vi "epics get uniformity.vi"(8 "error in":errorcluster, 11 "CA in":T2) -> (0 "error out":errorcluster, 1 "Status":bool, 2 "Values Out - String":string[](array[string]), 3 "Data Value Out":T3, 4 "PV Info":T1[](array[typedef]))   [LabVIEW 2022 SP3]
uses:
  Program Files/National Instruments/LabVIEW 2023/user.lib/calab/CaLab.lvlib
  Program Files/National Instruments/LabVIEW 2023/user.lib/calab/private/Get_PV.vi
  pectus/control/epics value.ctl
  271cf89c-c69d-42b5-ba05-be60b1157d68.vi
  pectus/control/ca cluster.ctl
  Program Files/National Instruments/LabVIEW 2023/user.lib/calab/PV Info.ctl
panel:
  out "Value out":variant
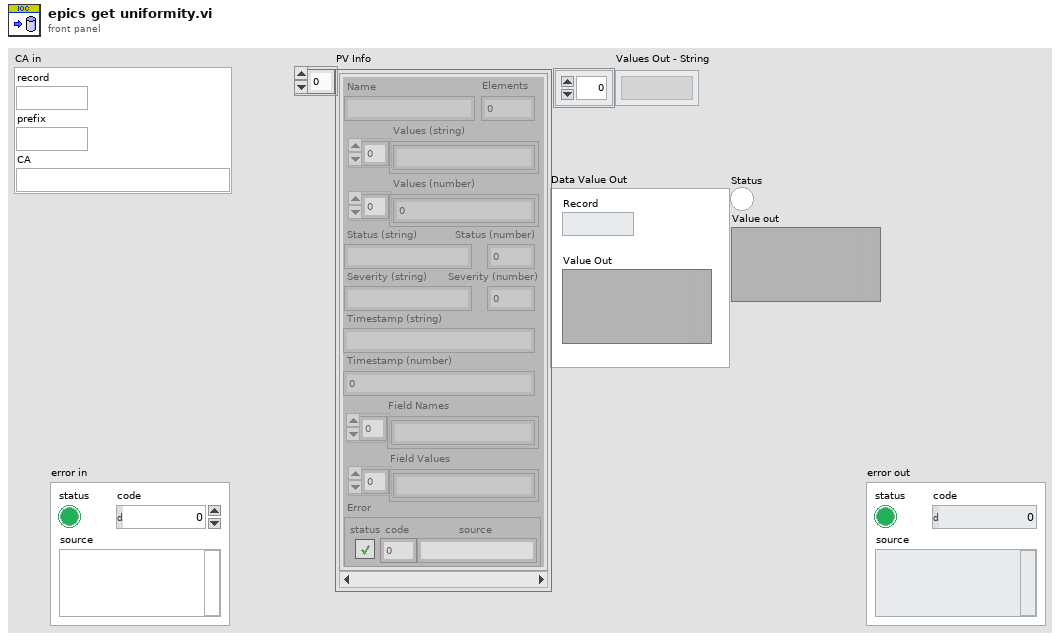
[diagram p1: front panel]
types:
  T1 = typedef "CaLab.lvlib/PV Info.ctl" = cluster{"Name":string, "Elements":i32, "Values (string)":string[], "Values (number)":dbl[], "Status (string)":string, "Status (number)":i16, "Severity (string)":string, "Severity (number)":i16, "Timestamp (string)":string, "Timestamp (number)":i32, "Field Names":string[], "Field Values":string[], "Error":errorcluster}
  T2 = typedef "ca cluster.ctl" = cluster{"record":string, "prefix":string, "CA":string}
  T3 = typedef "epics value.ctl" = cluster{"Record":string, "Value Out":variant}
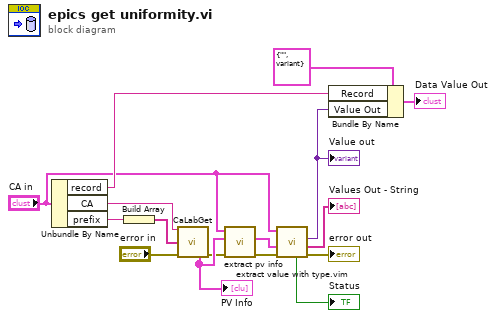
[diagram p0: block diagram]
diagram:
  n1 = Unbundle By Name("CA in") -> ("record"=w10:string, "CA"=w12:string, "prefix"=w11:string)
  n2 = Build Array(w11) -> (w16:string[])
  n3 = call-poly "CaLabGet.vi"("PV Name"=w12, "Field Names"=w16, "Error in (no error)"="error in") -> ("PV Info"=w8:T1[], "Error out"=w3:errorcluster)  [unwired: 6 in, 5 out]
  "PV Info" <- w8
  n4 = call "extract pv info.vi"("error in"=w3, "PV Info"=w8, "CA in"="CA in") -> ("error out"=w7:errorcluster, "PV Selected"=w6:T1)  [unwired: 7 in]
  n5 = call "extract value with type.vim"("error in"=w7, "PV Selected"=w6, "CA in"="CA in") -> ("error out"=→"error out":errorcluster, "Values Out - String"=→"Values Out - String":string[], "Value out"=w4:variant, "Status"=→"Status":bool)  [unwired: 5 in]
  "Value out" <- w4
  n6 = Bundle By Name(cluster=T3 {"Record"="", "Value Out"=variant} ("Data Out"), "Record"=w10, "Value Out"=w4) -> (→"Data Value Out":T3)
